vi "Begin.vi"(8 "error in":errorcluster) -> (0 "error out":errorcluster)   [LabVIEW 2020]
doc: "Called before other user functions, this VI is expected to open initial I/O refnums, load in file data, and do all program initialization. Notice that the <B>error out</B> terminal is simply used for data flow. Wiring it to other structures or subVIs ensures that this VI runs first."
uses:
  <vilib>/Rock Robotics/SystemInterfaces/DIO/FPGA_DIOPWMChannel.ctl
  Robot Global Data.vi
  <vilib>/Rock Robotics/WPI/DriverStation/WPI_DriverStationRobotMode2.ctl
  <vilib>/Rock Robotics/WPI/Joystick/WPI_JoystickDeviceEnum.ctl
  <vilib>/Rock Robotics/Network Tables/NT Write String Array.vi
  <vilib>/Rock Robotics/SystemInterfaces/AI/FPGA_AIChannel.ctl
  <vilib>/Rock Robotics/WPI/MotorControl/WPI_MotorControlOpen VictorSP.vi
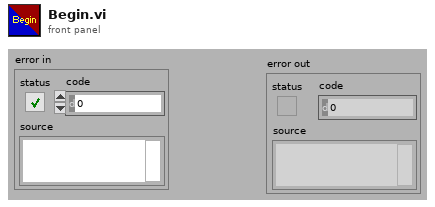
[diagram p1: front panel]
types:
  T1 = typedef "FPGA_AIChannel.ctl" = enum8{"AI 0", "AI 1", "AI 2", "AI 3", "AI MXP 0", "AI MXP 1", "AI MXP 2", "AI MXP 3", "Invalid"}
  T2 = cluster{"Pot. Voltage":dbl[], "Corresponding Inches":dbl[]}
  T3 = typedef "FPGA_DIOPWMChannel.ctl" = enum8{"PWM 0", "PWM 1", "PWM 2", "PWM 3", "PWM 4", "PWM 5", "PWM 6", "PWM 7", "PWM 8", "PWM 9", "PWM MXP 0", "PWM MXP 1", "PWM MXP 2", "PWM MXP 3", "PWM MXP 4", "PWM MXP 5", "PWM MXP 6", "PWM MXP 7", "PWM MXP 8", "PWM MXP 9", "Invalid"}
  T4 = typedef "WPI_JoystickDeviceEnum.ctl" = enum16{"USB 0", "USB 1", "USB 2", "USB 3", "USB 4", "USB 5"}
  T5 = typedef "WPI_DriverStationRobotMode2.ctl" = enum16{"Autonomous Disabled", "Autonomous Enabled", "Teleop Disabled", "Teleop Enabled", "Disconnected", "Finish", "Test Disabled", "Test Enabled", "Emergency Stopped"}
  T6 = typedef "WPI_MotorControlDeviceRef.ctl" = cluster{"DeviceStatus":errorcluster, "Type":T7, "PWM":cluster{"PWM Channel":T3, "DeadBand":T8}, "CAN":cluster{"Device Number":u8, "SetOutput VI Ref":variant, "GetOutput VI Ref":variant, "Enable VI Ref":variant, "Disable VI Ref":variant, "Data":variant}, "Invert":bool, "DIO PWM":cluster{"PWM \"Enable\" Channel":T3, "DIOChannel":T9, "PWM Rate":dbl}}
  T7 = typedef "WPI_MotorControlType.ctl" = enum16{"PWM", "CAN", "DIO PWM"}
  T8 = typedef "WPI_PWMDeadband.ctl" = cluster{"Name":string, "maxPositivePwm":i32, "minPositivePwm":i32, "centerPwm":i32, "maxNegativePwm":i32, "minNegativePwm":i32, "angularRange":u16}
  T9 = typedef "FPGA_DIOChannel.ctl" = enum8{"DIO 0", "DIO 1", "DIO 2", "DIO 3", "DIO 4", "DIO 5", "DIO 6", "DIO 7", "DIO 8", "DIO 9", "DIO MXP 0", "DIO MXP 1", "DIO MXP 2", "DIO MXP 3", "DIO MXP 4", "DIO MXP 5", "DIO MXP 6", "DIO MXP 7", "DIO MXP 8", "DIO MXP 9", "DIO MXP 10", "DIO MXP 11", "DIO MXP 12", "DIO MXP 13", "DIO MXP 14", "DIO MXP 15", "SPI Port CS1", "SPI Port CS2", "SPI Port CS3", "SPI Port MISO", "SPI Port MOSI", "Invalid"}
  T10 = typedef "WPI_ServoDeviceRef.ctl" = cluster{"DeviceStatus":errorcluster, "PWM Channel":T3, "DeadBand":T8}
  T11 = typedef "WPI_PotentiometerDevRef.ctl" = cluster{"DevStatus":errorcluster, "Analog Channel":T1, "Invert Output":bool}
  T12 = typedef "WPI_JoystickDevRef.ctl" = cluster{"Device":T4}
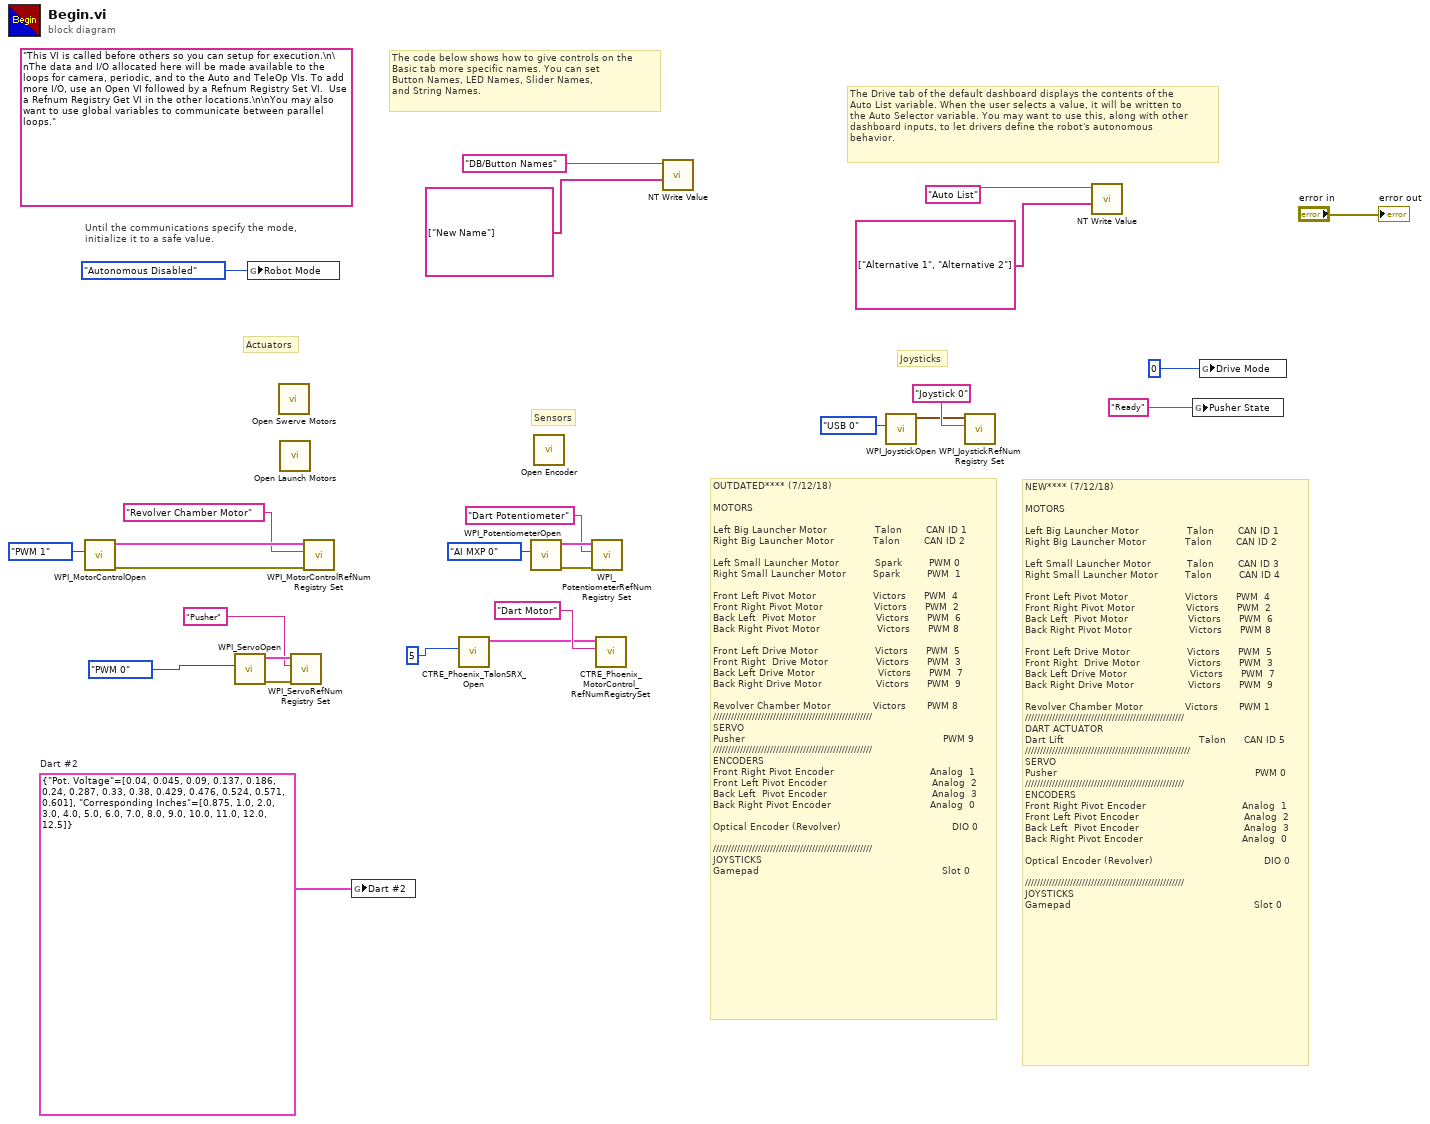
[diagram p0: block diagram]
diagram:
  w9 = T2 {"Pot. Voltage"=[0.04, 0.045, 0.09, 0.137, 0.186, 0.24, 0.287, 0.33, 0.38, 0.429, 0.476, 0.524, 0.571, 0.601], "Corresponding Inches"=[0.875, 1.0, 2.0, 3.0, 4.0, 5.0, 6.0, 7.0, 8.0, 9.0, 10.0, 11.0, 12.0, 12.5]}  # Dart #2
  (unwired) "This VI is called before others so you can setup for execution.\n\nThe data and I/O allocated here will be made available to the loops for camera, periodic, and to the Auto and TeleOp VIs. To add more I/O, use an Open VI followed by a Refnum Registry Set VI.  Use a Refnum Registry Get VI in the other locations.\n\nYou may also want to use global variables to communicate between parallel loops."
  # "NEW**** (7/12/18)\n\nMOTORS\n\nLeft Big Launcher Motor                Talon        CAN ID 1\nRight Big Launcher Motor             Talon        CAN ID 2\n\nLeft Small Launcher Motor            Talon        CAN ID 3\nRight Small Launcher Motor         Talon         CAN ID 4\n\nFront Left Pivot Motor                   Victors      PWM  4\nFront Right Pivot Motor                 Victors      PWM  2\nBack Left  Pivot Motor                    Victors      PWM  6\nBack Right Pivot Motor                   Victors      PWM 8\n \nFront Left Drive Motor                   Victors      PWM  5\nFront Right  Drive Motor                Victors      PWM  3\nBack Left Drive Motor                     Victors      PWM  7\nBack Right Drive Motor                  Victors      PWM  9\n\nRevolver Chamber Motor              Victors       PWM 1\n/////////////////////////////////////////////////////\nDART ACTUATOR\nDart Lift                                             Talon      CAN ID 5\n///////////////////////////////////////////////////////\nSERVO\nPusher                                                                  PWM 0\n/////////////////////////////////////////////////////\nENCODERS\nFront Right Pivot Encoder                                Analog  1\nFront Left Pivot Encoder                                   Analog  2\nBack Left  Pivot Encoder                                   Analog  3\nBack Right Pivot Encoder                                 Analog  0\n\nOptical Encoder (Revolver)                                     DIO 0\n\n/////////////////////////////////////////////////////\nJOYSTICKS\nGamepad                                                             Slot 0"
  # "OUTDATED**** (7/12/18)\n\nMOTORS\n\nLeft Big Launcher Motor                Talon        CAN ID 1\nRight Big Launcher Motor             Talon        CAN ID 2\n\nLeft Small Launcher Motor            Spark         PWM 0\nRight Small Launcher Motor         Spark         PWM  1\n\nFront Left Pivot Motor                   Victors      PWM  4\nFront Right Pivot Motor                 Victors      PWM  2\nBack Left  Pivot Motor                    Victors      PWM  6\nBack Right Pivot Motor                   Victors      PWM 8\n \nFront Left Drive Motor                   Victors      PWM  5\nFront Right  Drive Motor                Victors      PWM  3\nBack Left Drive Motor                     Victors      PWM  7\nBack Right Drive Motor                  Victors      PWM  9\n\nRevolver Chamber Motor              Victors       PWM 8\n/////////////////////////////////////////////////////\nSERVO\nPusher                                                                  PWM 9\n/////////////////////////////////////////////////////\nENCODERS\nFront Right Pivot Encoder                                Analog  1\nFront Left Pivot Encoder                                   Analog  2\nBack Left  Pivot Encoder                                   Analog  3\nBack Right Pivot Encoder                                 Analog  0\n\nOptical Encoder (Revolver)                                     DIO 0\n\n/////////////////////////////////////////////////////\nJOYSTICKS\nGamepad                                                             Slot 0"
  # "Sensors"
  # "Actuators"
  # "Joysticks"
  # "The Drive tab of the default dashboard displays the contents of the\nAuto List variable. When the user selects a value, it will be written to\nthe Auto Selector variable. You may want to use this, along with other\ndashboard inputs, to let drivers define the robot's autonomous\nbehavior."
  # "The code below shows how to give controls on the\nBasic tab more specific names. You can set\nButton Names, LED Names, Slider Names,\nand String Names."
  # "Until the communications specify the mode,\ninitialize it to a safe value."
  n1 = call-poly <vilib>:"WPI_MotorControlOpen.vi"("PWM Channel"=FPGA_DIOPWMChannel."PWM 1") -> ("error out"=w13:errorcluster, "MotorControlDeviceRef"=w14:T6)  [unwired: 9 in]
  n2 = call <vilib>:"WPI_ServoOpen.vi"("PWM Channel"=FPGA_DIOPWMChannel."PWM 0") -> ("error out"=w18:errorcluster, "ServoDeviceRef"=w17:T10)  [unwired: 9 in]
  n3 = global write "Robot Global Data.vi" "Robot Mode"(WPI_DriverStationRobotMode2."Autonomous Disabled" ("Robot Mode")) -> ()
  n4 = call "Open Swerve Motors.vi"() -> ()  [unwired: 12 in]
  n5 = call "Open Launch Motors.vi"() -> ()  [unwired: 8 in, 4 out]
  n6 = call <vilib>:"WPI_ServoRefNum Registry Set.vi"("error in (no error)"=w18, "refnum name"="Pusher", "ServoDeviceRef"=w17) -> ()  [unwired: 7 in, 2 out]
  n7 = call <vilib>:"WPI_MotorControlRefNum Registry Set.vi"("error in (no error)"=w13, "refnum name"="Revolver Chamber Motor", "MotorControlDevRef"=w14) -> ()  [unwired: 7 in, 2 out]
  n8 = global write "Robot Global Data.vi" "Dart #2"(w9) -> ()
  n9 = call <vilib>:"CTRE_Phoenix_TalonSRX_Open.vi"("Device Number"=5) -> ("PhoenixMotorControlDevRef"=w2:T6)  [unwired: 9 in, 1 out]
  n10 = call <vilib>:"WPI_PotentiometerOpen.vi"("Analog Channel"=FPGA_AIChannel."AI MXP 0") -> ("error out"=w7:errorcluster, "PotDevRef"=w6:T11)  [unwired: 9 in]
  n11 = call "Open Encoder.vi"() -> ()  [unwired: 12 in]
  n12 = call <vilib>:"WPI_PotentiometerRefNum Registry Set.vi"("error in (no error)"=w7, "refnum name"="Dart Potentiometer", "PotDevRef"=w6) -> ()  [unwired: 7 in, 2 out]
  n13 = call <vilib>:"CTRE_Phoenix_MotorControl_RefNumRegistrySet.vi"("refnum name"="Dart Motor", "PhoenixMotorControlDevRef"=w2) -> ()  [unwired: 8 in, 2 out]
  n14 = call-poly <vilib>:"NT Write Value.vi"("value"=string[] ["New Name"], "name"="DB/Button Names" ("Name")) -> ()  [unwired: 9 in, 1 out]
  n15 = call <vilib>:"WPI_JoystickOpen.vi"("JoystickDevice"=WPI_JoystickDeviceEnum."USB 0") -> ("JoystickDevRef"=w25:T12)  [unwired: 10 in]
  n16 = call <vilib>:"WPI_JoystickRefNum Registry Set.vi"("refnum name"="Joystick 0", "JoystickDevRef"=w25) -> ()  [unwired: 8 in, 2 out]
  n17 = call-poly <vilib>:"NT Write Value.vi"("value"=string[] ["Alternative 1", "Alternative 2"] ("String Array"), "name"="Auto List" ("Name")) -> ()  [unwired: 9 in, 1 out]
  n18 = global write "Robot Global Data.vi" "Pusher State"("Ready") -> ()
  n19 = global write "Robot Global Data.vi" "Drive Mode"(0) -> ()
  "error out" <- "error in"
